vi "Field Draw Future Robot.vi"(4 "Lado":enum16{"Esquerdo", "Direito"}(ring) caption="Enum", 6 "Draw Targets?":T1, 8 "Scale mm/pixel":dbl, 9 "Offset":T5, 10 "Robot":T2={"id"=0, "function"=enum."Attacker", "x"=0.0, "y"=0.0, "orientation"=0.0, "v_tangent"=0.0, "v_normal"=0.0, "v_ang"=0.0, "kick_x"=0.0, "kick_z"=0.0, "dribble"=FALSE, "Timestamp"=timestamp(0 s since 1904-01-01), "dest_x"=0.0, "dest_y"=0.0, "dest_orientation"=0.0, "estimatives"={"est_v_tangent"=0.0, "est_v_normal"=0.0, "est_vx"=0.0, "est_vy"=0.0, "Pos Robot Est"=[]}, "dest_x_kick"=0.0, "dest_y_kick"=0.0, "Gap Coord"=[], "States"=enum."GoToTangent"}, 11 "picture in":picture) -> (2 "picture out":picture)   [LabVIEW 2017]
uses:
  <vilib>/Utility/miscctls.llb/LVBoundsTypeDef.ctl
  Core/AI Robot.ctl
  Intel/Functions Enum.ctl
  Intel/AttackerStates.ctl
  DrawTargets.ctl
  <vilib>/Analysis/NI_AALPro.lvlib
  <vilib>/Analysis/coordinate.llb/2D Cartesian Coordinate Rotation (Scalar).vi
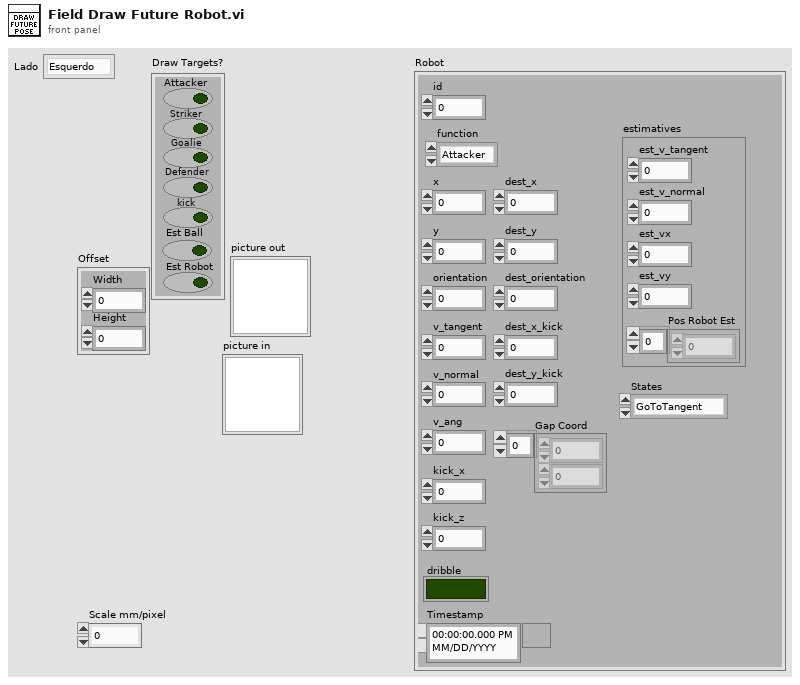
[diagram p1: front panel]
types:
  T1 = typedef "DrawTargets.ctl" = cluster{"Attacker":bool, "Striker":bool, "Goalie":bool, "Defender":bool, "kick":bool, "Est Ball":bool, "Est Robot":bool}
  T2 = typedef "AI Robot.ctl" = cluster{"id":u32, "function":T3, "x":dbl, "y":dbl, "orientation":dbl, "v_tangent":dbl, "v_normal":dbl, "v_ang":dbl, "kick_x":dbl, "kick_z":dbl, "dribble":bool, "Timestamp":timestamp, "dest_x":dbl, "dest_y":dbl, "dest_orientation":dbl, "estimatives":cluster{"est_v_tangent":dbl, "est_v_normal":dbl, "est_vx":dbl, "est_vy":dbl, "Pos Robot Est":dbl[]}, "dest_x_kick":dbl, "dest_y_kick":dbl, "Gap Coord":dbl[], "States":T4}
  T3 = typedef "Functions Enum.ctl" = enum16{"Attacker", "Goalie", "Defender", "Striker", "Goto 0", "Dummy", "Kicker", "ZigZag"}
  T4 = typedef "AttackerStates.ctl" = enum16{"Pass", "GoToTangent", "BallGetting", "GoToKick", ""}
  T5 = typedef "LVBoundsTypeDef.ctl" = cluster{"Width":u32, "Height":u32}
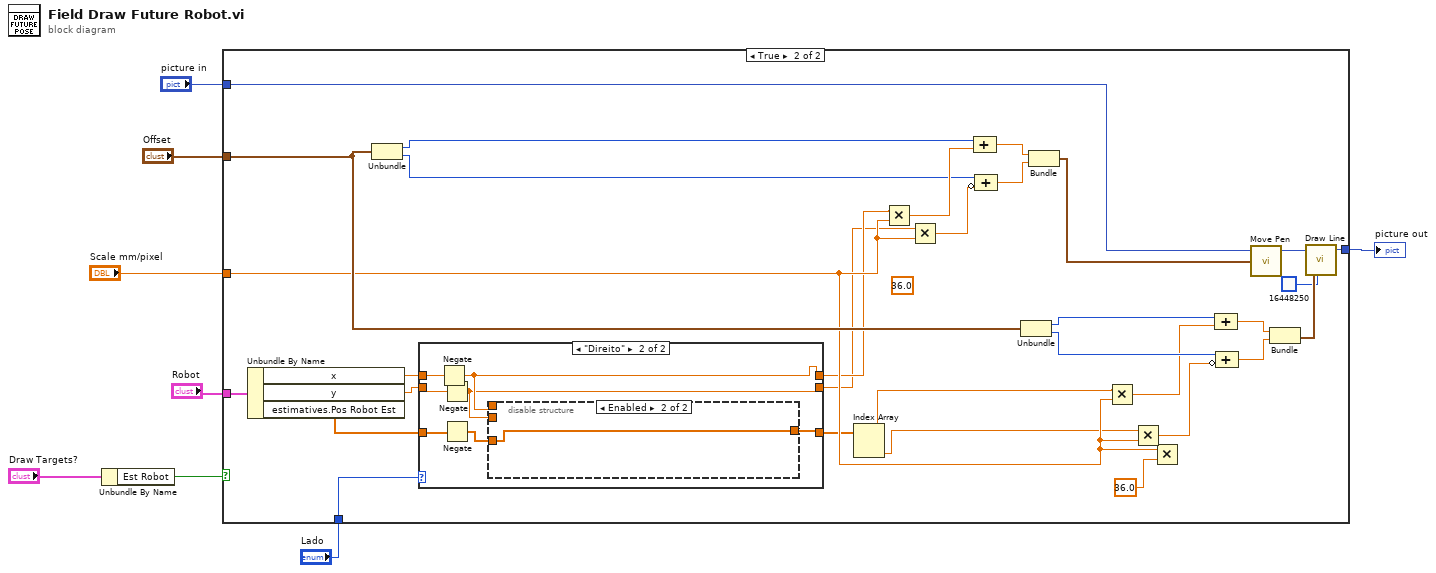
[diagram p0: block diagram]
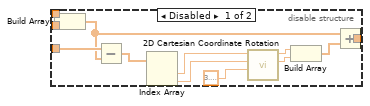
[diagram p4: hidden frame]
diagram:
  n1 = Unbundle By Name("Draw Targets?") -> ("Est Robot"=w2:bool)
  n2 = case shown="True" w2 {
    tunnel: [w9 w34] -> w8
    tunnel: "Offset" -> [_ w28]
    tunnel: "Scale mm/pixel" -> [_ w25]
    tunnel: "Robot" -> [_ w19]
    tunnel: "picture in" -> [w9 w18]
    tunnel: "Lado" -> [_ w16]
    frame False {
    }
    frame True {
      (unwired) sgl 36.0 ("radius")
      n3 = Unbundle By Name(w19) -> ("x"=w15:dbl, "y"=w13:dbl, "estimatives.Pos Robot Est"=w11:dbl[])
      n4 = Unbundle(w28) -> ("Width"=w40:u32, "Height"=w37:u32)
      n5 = case shown="\"Direito\"" w16 {
        tunnel: [w43 w47] -> w14
        tunnel: w15 -> [w43 w50]
        tunnel: [w42 w46] -> w12
        tunnel: w13 -> [w42 w49]
        tunnel: [w41 w44] -> w10
        tunnel: w11 -> [w41 w48]
        frame "Esquerdo", Default {
        }
        frame "Direito" {
          n6 = Negate(x=w50) -> (-x=w47:dbl)
          n7 = Negate(x=w49) -> (-x=w46:dbl)
          n8 = Negate(x=w48) -> (-x=w45:dbl[])
          n9 = disable-structure shown="Enabled" {
            disable-tunnel: w47 -> [w57 _]
            disable-tunnel: w46 -> [w56 _]
            disable-tunnel: w45 -> [w55 w63]
            disable-tunnel: [w53 w63] -> w44
            frame Disabled {
              n10 = Build Array(w57, w56) -> (w51:dbl[])
              n11 = Subtract(x=w55, y=w51) -> (x-y=w54:dbl[])
              n12 = Index Array(array=w54) -> (element #1=w62:dbl, element #2=w61:dbl)  [unwired: 2 in]
              n13 = call-poly <vilib>:"2D Cartesian Coordinate Rotation.vi"("theta"=3.141592653589793, "y"=w61, "x"=w62) -> ("y out"=w59:dbl, "x out"=w60:dbl)  [unwired: 6 in, 1 out]
              n14 = Build Array(w60, w59) -> (w52:dbl[])
              n15 = Add(x=w51, y=w52) -> (x+y=w53:dbl[])
            }
            frame Enabled {
            }
          }
        }
      }
      n16 = Index Array(array=w10) -> (element #1=w22:dbl, element #2=w21:dbl)  [unwired: 2 in]
      n17 = Multiply(x=w14, y=w25) -> (x*y=w39:dbl)
      n18 = Multiply(x=w12, y=w25) -> (x*y=w36:dbl)
      n19 = Compound Arithmetic op=ADD(w40, w39) -> (w38:dbl)
      n20 = Compound Arithmetic op=ADD(w37, invert w36) -> (w35:dbl)
      n21 = Unbundle(w28) -> ("Width"=w32:u32, "Height"=w30:u32)
      n22 = Bundle(w38, w35) -> (w17:cluster{dbl, dbl})  [unwired: 1 in]
      n23 = Multiply(x=w22, y=w25) -> (x*y=w24:dbl)
      n24 = Multiply(x=w21, y=w25) -> (x*y=w23:dbl)
      n25 = Multiply(x=w25, y=sgl 36.0 ("radius")) -> ()  [unwired: 1 out]
      n26 = Compound Arithmetic op=ADD(w32, w24) -> (w31:dbl)
      n27 = Compound Arithmetic op=ADD(w30, invert w23) -> (w29:dbl)
      n28 = call <vilib>:"Move Pen.vi"("new position"=w17, "picture"=w18) -> ("new picture"=w33:picture)  [unwired: 3 in]
      n29 = Bundle(w31, w29) -> (w27:cluster{dbl, dbl})  [unwired: 1 in]
      n30 = call <vilib>:"Draw Line.vi"("picture"=w33, "end point"=w27, "color(black)"=u32 16448250) -> ("new picture"=w34:picture)  [unwired: 6 in]
    }
  }
  "picture out" <- w8
